vi "PinkNoiseGen.vi"() -> ()   [LabVIEW 2014]
uses:
  <vilib>/sound/lvsound.llb/Sound Format.ctl
  <vilib>/Analysis/3filter.llb/IIR Filter (DBL).vi
  <vilib>/measure/maspectr.llb/Frequency Response Function (Mag-Phase) 1-1.vi
  <vilib>/Analysis/NI_AALBase.lvlib
  <vilib>/measure/NI_MAPro.lvlib
panel:
  in  "stop":bool
  in  "Sound Volume":u16(slide) scale=0.0..65535.0
  in  "White or Pink":bool
  in  "Play Noise?":bool
  in  "Sampling Rate":enum16{"8000", "11025", "22050", "44100"}(ring)
  in  "Filter Window":T1(ring)=enum."Hanning"
  in  "view":T2
  in  "averaging parameters":T3={"averaging mode"=enum."No averaging", "weighting mode"=enum."Exponential", "number of averages"=10} {"number of averages" min=1}
  in  "Reverse IIR Filter Coefficients":dbl[](array[numeric])=[-0.22231814100199035, 1.7211909155472194, -4.822432684064294, 6.3705074734613305, -4.0469475, 1.0] format="%.2f"
  in  "Forward IIR Filter Coefficients":dbl[](array[numeric])=[0.017693157210501197, 0.4607539307914841, -2.442774196843088, 4.43166582114909, -3.4673362, 1.0] format="%.2f"
  out "Frequency Response Function":cluster{"f0":dbl, "df":dbl, "magnitude":dbl[]}(graph)={"f0"=0.0, "df"=4.41, "magnitude"=array[5000 elements]}
  out "Noise Signal":waveform(dbl)(graph)={"t0"=timestamp(0 s since 1904-01-01), "dt"=2.2675736961451248e-05, "Y"=array[10000 elements]}
  # "Pink"
  # "White"
  # "These coefficients provide a -10 db/decade filter"
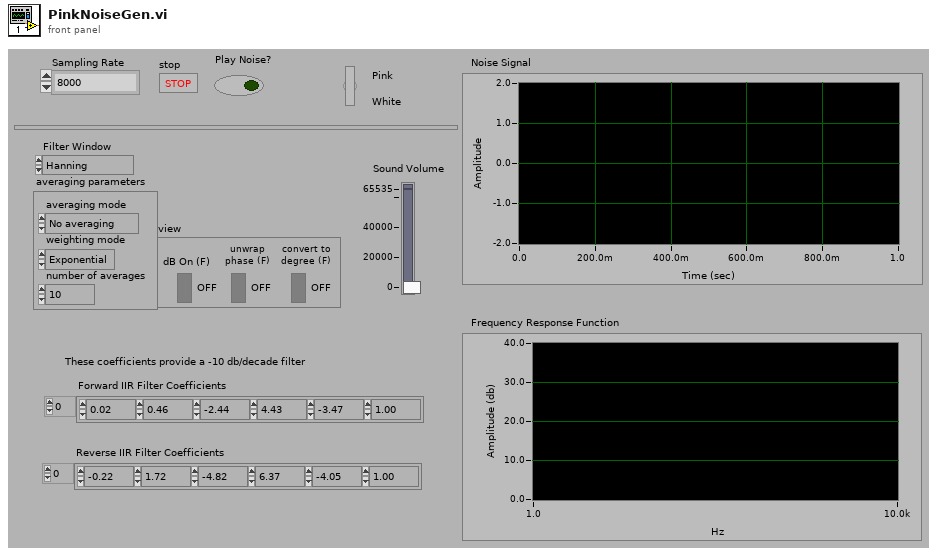
[diagram p1: front panel]
types:
  T1 = enum16{"None ", "Hanning", "Hamming", "Blackman-Harris", "Exact Blackman", "Blackman", "Flat Top", "4 Term B-Harris ", "7 Term B-Harris", "Low Sidelobe"}
  T2 = cluster{"dB On (F)":bool, "unwrap phase (F)":bool, "convert to degree (F)":bool}
  T3 = cluster{"averaging mode":enum16{"No averaging", "Vector averaging", "RMS averaging"}, "weighting mode":enum16{"Linear", "Exponential"}, "number of averages":u32}
  T4 = typedef "Sound Format.ctl" = cluster{"sound quality":enum16{"mono", "stereo"}, "rate":enum16{"11025", "22050", "44100", "8000"}, "bits per sample":enum16{"8 bit", "16 bit"}}
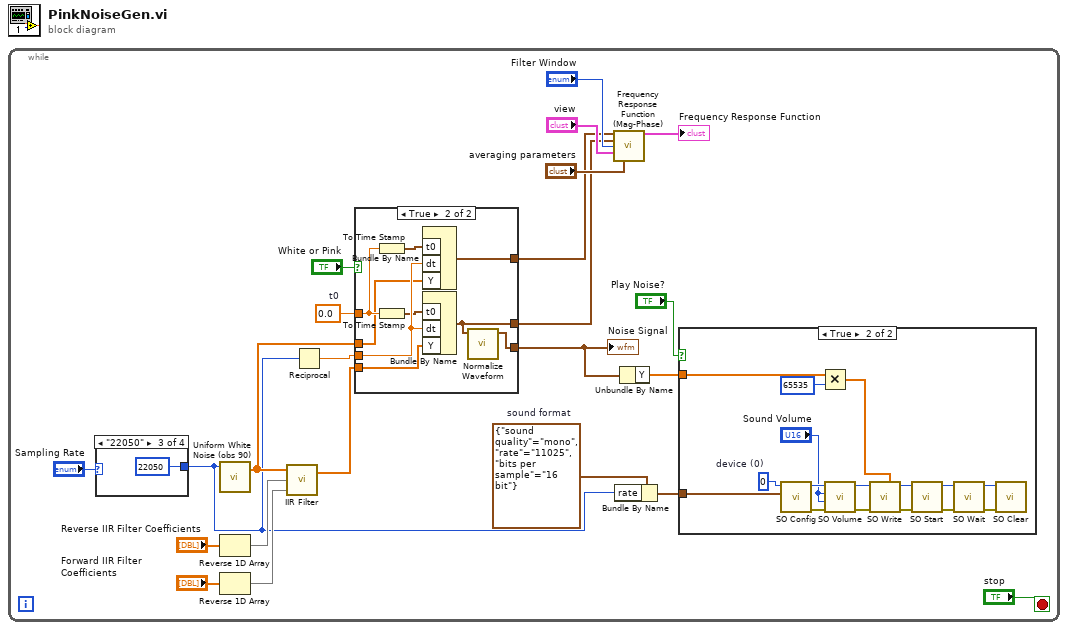
[diagram p0: block diagram]
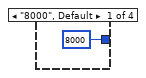
[diagram p3: hidden frame]
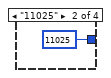
[diagram p4: hidden frame]
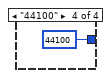
[diagram p5: hidden frame]
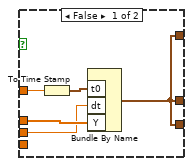
[diagram p6: hidden frame]
diagram:
  n1 = while {
    stop <- "stop" stop-if-true
    w6 = T4 {"sound quality"=enum."mono", "rate"=enum."11025", "bits per sample"=enum."16 bit"}  # sound format
    w19 = 0.0  # t0
    n2 = case shown="\"22050\"" "Sampling Rate" {
      tunnel: [8000 11025 i16 22050 44100] -> w5
      frame "8000", Default {
      }
      frame "11025" {
      }
      frame "22050" {
      }
      frame "44100" {
      }
    }
    n3 = call <vilib>:"Uniform White Noise (obs 90).vi"("samples"=w5) -> ("uniform white noise"=w10:dbl[])  [unwired: 2 in, 1 out]
    n4 = Reverse 1D Array(array="Reverse IIR Filter Coefficients") -> (reversed array=w20:dbl[])
    n5 = Reverse 1D Array(array="Forward IIR Filter Coefficients") -> (reversed array=w21:dbl[])
    n6 = call-poly <vilib>:"IIR Filter.vi"("Forward Coefficients"=w21, "Reverse Coefficients"=w20, "X"=w10) -> ("Filtered X"=w13:dbl[])  [unwired: 1 in, 1 out]
    n7 = Reciprocal(x=w5) -> (1/x=w17:dbl)
    n8 = case shown="True" "White or Pink" {
      tunnel: w19 -> [w46 w56]
      tunnel: w17 -> [w47 w55]
      tunnel: w13 -> [_ w57]
      tunnel: [w45 w52] -> w11
      tunnel: w10 -> [w48 w54]
      tunnel: [w45 w51] -> w3
      tunnel: [w45 w53] -> w9
      frame False {
        n9 = To Time Stamp(1:w46) -> (0:w44:timestamp)
        n10 = Bundle By Name("t0"=w44, "dt"=w47, "Y"=w48) -> (w45:waveform(dbl))  [unwired: 1 out]
      }
      frame True {
        n11 = To Time Stamp(1:w56) -> (0:w50:timestamp)
        n12 = To Time Stamp(1:w56) -> (0:w49:timestamp)
        n13 = Bundle By Name("t0"=w50, "dt"=w55, "Y"=w54) -> (w53:waveform(dbl))  [unwired: 1 out]
        n14 = Bundle By Name("t0"=w49, "dt"=w55, "Y"=w57) -> (w52:waveform(dbl))  [unwired: 1 out]
        n15 = call <vilib>:"Normalize Waveform.vi"("waveform in"=w52) -> ("normalized waveform"=w51:waveform(dbl))  [unwired: 2 in, 8 out]
      }
    }
    "Noise Signal" <- w3
    n16 = call-poly <vilib>:"Frequency Response Function (Mag-Phase).vi"("time signal X"=w9, "time signal Y"=w11, "window"="Filter Window", "view"="view", "averaging parameters"="averaging parameters") -> ("magnitude"=→"Frequency Response Function":cluster{"f0":dbl, "df":dbl, "magnitude":dbl[]})  [unwired: 3 in, 7 out]
    n17 = Bundle By Name(cluster=w6, "rate"=w5) -> (w4:T4)
    n18 = Unbundle By Name(w3) -> ("Y"=w2:dbl[])
    n19 = case shown="True" "Play Noise?" {
      tunnel: w4 -> [_ w32]
      tunnel: w2 -> [_ w31]
      frame False {
      }
      frame True {
        w33 = u32 0  # device (0)
        n20 = call <vilib>:"SO Config.vi"("sound format"=w32, "device (0)"=w33) -> ("error out"=w27:errorcluster, "task ID out"=w28:u32)  [unwired: 1 in, 7 out]
        n21 = Multiply(x=w31, y=65535) -> (x*y=w29:dbl[])
        n22 = call <vilib>:"SO Volume.vi"("error in (no error)"=w27, "right channel"="Sound Volume", "left channel"="Sound Volume", "task ID in"=w28) -> ("error out"=w26:errorcluster, "task ID out"=w25:u32)  [unwired: 6 out]
        n23 = call <vilib>:"SO Write.vi"("mono 16-bit"=w29, "error in (no error)"=w26, "task ID in"=w25) -> ("error out"=w39:errorcluster, "task ID out"=w38:u32)  [unwired: 3 in, 4 out]
        n24 = call <vilib>:"SO Start.vi"("error in (no error)"=w39, "task ID in"=w38) -> ("error out"=w37:errorcluster, "task ID out"=w36:u32)  [unwired: 8 out]
        n25 = call <vilib>:"SO Wait.vi"("error in (no error)"=w37, "task ID in"=w36) -> ("error out"=w35:errorcluster, "task ID out"=w34:u32)  [unwired: 8 out]
        n26 = call <vilib>:"SO Clear.vi"("error in (no error)"=w35, "task ID in"=w34) -> ()  [unwired: 10 out]
      }
    }
  }
